vi "assemble.vi"(8 "error in (no error)":errorcluster, 11 "Chair in":refnum<class "Chair.lvclass">) -> (0 "error out":errorcluster, 2 "String":string="assembeld", 3 "Chair out":refnum<class "Chair.lvclass">)   [LabVIEW 2021, in "Chair.lvclass"]
uses:
  Chair.lvclass
  Chair.lvclass/Chair.ctl
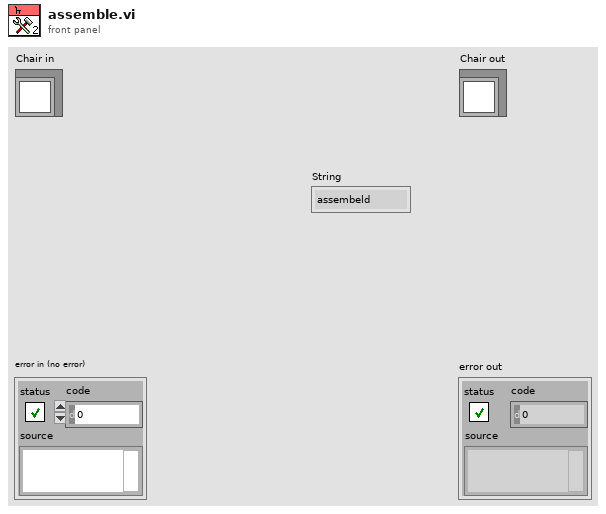
[diagram p1: front panel]
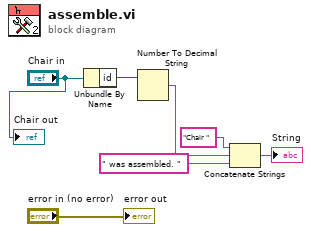
[diagram p0: block diagram]
diagram:
  n1 = Unbundle By Name("Chair in") -> ("id"=w2:u32)
  n2 = Number To Decimal String(number=w2) -> (decimal integer string=w1:string)  [unwired: 1 in]
  n3 = Concatenate Strings("Chair ", w1, " was assembled. ") -> (→"String":string)
  "error out" <- "error in (no error)"
  "Chair out" <- "Chair in"
